vi "Get Command Infos.vi"(8 "error in (no error)":errorcluster, 11 "Keyboard in":refnum<class "Keyboard.lvclass">) -> (0 "error out":errorcluster, 3 "Keyboard out":refnum<class "Keyboard.lvclass">, 4 "Direction info out":string, 6 "Boost info out":string)   [LabVIEW 2021, in "Keyboard.lvclass"]
doc: "MIT Licence\nCopyright (c) 2024 David Grollier"
uses:
  Keyboard.lvclass
  Keyboard.lvclass/Keyboard.ctl
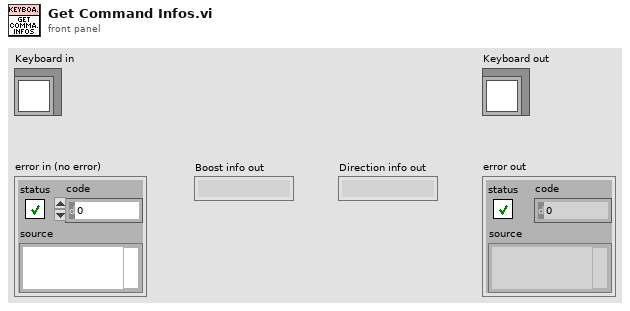
[diagram p1: front panel]
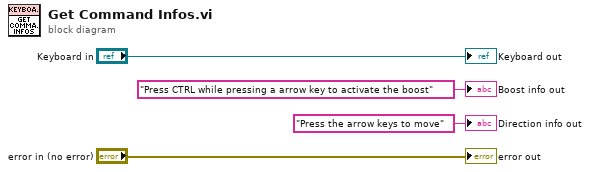
[diagram p0: block diagram]
diagram:
  "error out" <- "error in (no error)"
  "Keyboard out" <- "Keyboard in"
  "Direction info out" <- "Press the arrow keys to move" ("Direction info out")
  "Boost info out" <- "Press CTRL while pressing a arrow key to activate the boost" ("Boost info out")
